vi "Sys config window-Hide redundant ctrls.vi"(8 "error in (no error)":errorcluster, 10 "MC Visible?":bool, 11 "Pos ctrl window refs":T1) -> (0 "error out":errorcluster)   [LabVIEW 2020]
uses:
  Typedefs/HW config window refs cluster.ctl
  Typedefs/HW Setup tab control.ctl
  Typedefs/Control Sys HW config cluster.ctl
  Typedefs/CTRL system config.ctl
  Peripherals Control/Triggers/Typedefs/General trigger settings cluster.ctl
  Typedefs/Trigger 1 selector enum.ctl
  Typedefs/Triggers HW config.ctl
  Peripherals Control/Triggers/Typedefs/Triggers output setup.ctl
  Peripherals Control/Triggers/Typedefs/Trigger setup element cluster.ctl
  Typedefs/DAQ FPGA HW config cluster.ctl
  RIG-SPECIFIC FILES/FPGA Refs/FPGA Ref.ctl
  <vilib>/userDefined/High Color/nirio_resource_hc.ctl
  Typedefs/FPGA input type AC-DC.ctl
  Typedefs/DAQ FPGA system config.ctl
  Peripherals Control/XYZ Stage/Control/typedefs/XYZControlConfig.ctl
  Typedefs/Peripherals comms config cluster.ctl
  Typedefs/Comms Type.ctl
  Typedefs/Encoder config cluster.ctl
  Typedefs/Cam VidRec HW config setup cluster.ctl
  Typedefs/AOD Settings-distilled.ctl
  Typedefs/Laser Power Control HW config.ctl
  Typedefs/Laser 1 config cluster.ctl
  Typedefs/PreChirper 1 config cluster.ctl
  Typedefs/PreChirper constants.ctl
panel:
  # "General Setup"
  # "Control System"
  # "Triggers"
  # "DAQ FPGA"
  # "HW Channels Setup"
  # "XYZ Stage"
  # "Encoder"
  # "redundant"
  # "redundant"
  # "redundant"
  # "redundant"
  # "Hardware Setup"
  # "CamVideo"
  # "redundant"
  # "redundant"
  # "AOL Properties"
  # "Calib. Settings"
  # "Laser Settings"
  # "PreChirper Settings"
  # "(make , model etc)"
  # "(COM Port / IP Address / service address etc.)"
  # "(Port for ethernet / channel for BT)"
  # "(make , model etc)"
  # "(COM Port / IP Address / service address etc.)"
  # "(Port for ethernet / channel for BT)"
  # "(make , model etc)"
  # "(COM Port / IP Address / service address etc.)"
  # "(Port for ethernet / channel for BT)"
  # "Thickness (mm)"
  # "X Offset"
  # "Separation (mm)"
  # "Y Offset"
  # "Centre (mm)"
  # "Timing Offset"
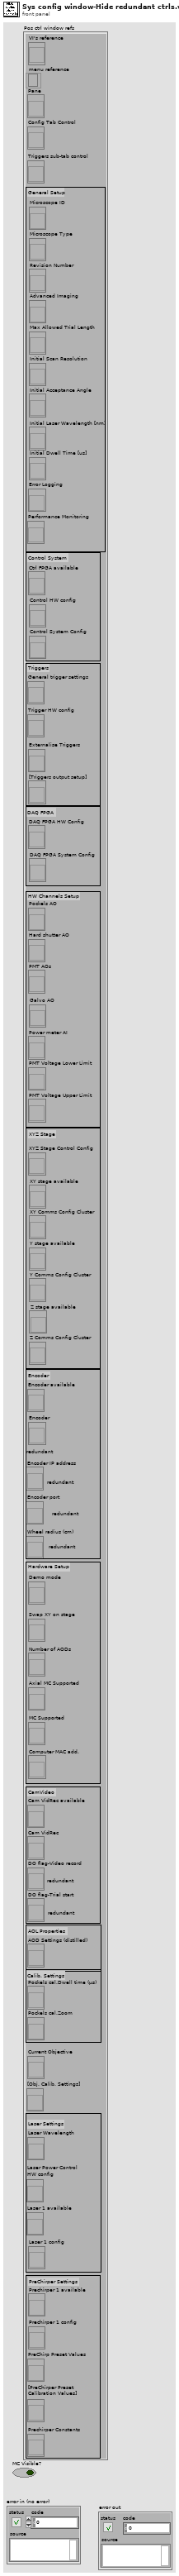
[diagram p1: front panel]
types:
  T1 = typedef "HW config window refs cluster.ctl" = cluster{"VI's reference":refnum<vi>, "menu reference":refnum<k9>, "Pane":refnum<vi>, "Config Tab Control":refnum<vi>, "Triggers sub-tab control":refnum<vi>, "Microscope ID":refnum<vi>, "Microscope Type":refnum<vi>, "Revision Number":refnum<vi>, "Advanced Imaging":refnum<vi>, "Max Allowed Trial Length":refnum<vi>, "Initial Scan Resolution":refnum<vi>, "Initial Acceptance Angle":refnum<vi>, "Initial Laser Wavelength [nm] ":refnum<vi>, "Initial Dwell Time [us]":refnum<vi>, "Error Logging":refnum<vi>, "Performance Monitoring":refnum<vi>, "Ctrl FPGA available":refnum<vi>, "Control HW config":refnum<vi>, "Control System Config":refnum<vi>, "General trigger settings":refnum<vi>, "Trigger HW config":refnum<vi>, "Externalise Triggers":refnum<vi>, "[Triggers output setup]":refnum<vi>, "DAQ FPGA HW Config":refnum<vi>, "DAQ FPGA System Config":refnum<vi>, "Pockels AO":refnum<vi>, "Hard shutter AO":refnum<vi>, "PMT AOs":refnum<vi>, "Galvo AO":refnum<vi>, "Power meter AI":refnum<vi>, "PMT Voltage Lower Limit":refnum<vi>, "PMT Voltage Upper Limit":refnum<vi>, "XYZ Stage Control Config":refnum<vi>, "XY stage available":refnum<vi>, "XY Comms Config Cluster":refnum<vi>, "Y stage available":refnum<vi>, "Y Comms Config Cluster":refnum<vi>, "Z stage available":refnum<vi>, "Z Comms Config Cluster":refnum<vi>, "Encoder available":refnum<vi>, "Encoder":refnum<vi>, "Encoder IP address":refnum<vi>, "Encoder port":refnum<vi>, "Wheel radius (cm)":refnum<vi>, "Demo mode":refnum<vi>, "Swap XY on stage":refnum<vi>, "Number of AODs":refnum<vi>, "Axial MC Supported":refnum<vi>, "MC Supported":refnum<vi>, "Computer MAC add.":refnum<vi>, "Cam VidRec available":refnum<vi>, "Cam VidRec":refnum<vi>, "DO flag-Video record":refnum<vi>, "DO flag-Trial start":refnum<vi>, "AOD Settings (distilled)":refnum<vi>, "Pockels cal.Dwell time (µs)":refnum<vi>, "Pockels cal.Zoom":refnum<vi>, "Current Objective":refnum<vi>, "[Obj. Calib. Settings]":refnum<vi>, "Laser Wavelength":refnum<vi>, "Laser Power Control \nHW config":refnum<vi>, "Laser 1 available":refnum<vi>, "Laser 1 config":refnum<vi>, "Prechirper 1 available":refnum<vi>, "Prechirper 1 config":refnum<vi>, "PreChirp Preset Values":refnum<vi>, "[PreChirper Preset \nCalibration Values]":refnum<vi>, "Prechirper Constants":refnum<vi>}
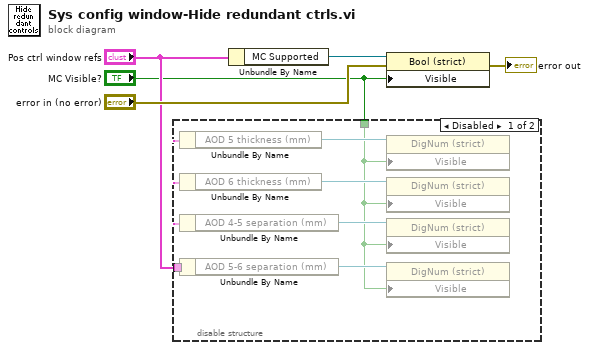
[diagram p0: block diagram]
diagram:
  n1 = disable-structure shown="Disabled" {
    disable-tunnel: "Pos ctrl window refs" -> [w7 _]
    disable-tunnel: "MC Visible?" -> [w6 _]
    frame Disabled {
      n2 = Unbundle By Name(w7) -> ("AOD 5 thickness (mm)"=w11:refnum<vi>)
      n3 = Unbundle By Name(w7) -> ("AOD 6 thickness (mm)"=w10:refnum<vi>)
      n4 = Unbundle By Name(w7) -> ("AOD 4-5 separation (mm)"=w9:refnum<vi>)
      n5 = Unbundle By Name(w7) -> ("AOD 5-6 separation (mm)"=w8:refnum<vi>)
      n6 = property on="Property Node" class="DigNum (strict)"(reference=w11, "Visible"=w6) -> ()  [unwired: 1 in, 2 out]
      n7 = property on="Property Node" class="DigNum (strict)"(reference=w10, "Visible"=w6) -> ()  [unwired: 1 in, 2 out]
      n8 = property on="Property Node" class="DigNum (strict)"(reference=w9, "Visible"=w6) -> ()  [unwired: 1 in, 2 out]
      n9 = property on="Property Node" class="DigNum (strict)"(reference=w8, "Visible"=w6) -> ()  [unwired: 1 in, 2 out]
    }
    frame Enabled {
    }
  }
  n10 = Unbundle By Name("Pos ctrl window refs") -> ("MC Supported"=w3:refnum<vi>)
  n11 = property on="Property Node" class="Bool (strict)"(reference=w3, error in="error in (no error)", "Visible"="MC Visible?") -> (error out=→"error out":errorcluster)  [unwired: 1 out]
